vi "Build New AIM ARINC 664 Custom Device.vi"(6 "Bin File Parameter Data":path=path "Support/2FrameProperlyDefined.bin", 7 "Base System Definition File":path=path "Support/Base.nivssdf", 9 "XML File Parameter Data":path=path "Support/UDP_RX_TX_Loopback_TxRxMon.xml", 11 "Output System Definition File":path=path "Support/Scripted AIM ARINC 664.nivssdf") -> (3 "AIM ARINC 664 System Definition":path)   [LabVIEW 2020]
doc: "Overview: Demonstrates using the AIM ARINC 664 scripting API to configure the custom device by building from configuration clusters. \n\nInstructions:\n1. Run this example VI, which will create an instance of the AIM ARINC 664 Custom Device in a VeriStand system definition with a configuration matching the constants on the block diagram.\n2. (VeriStand) Optionally, you may open the Output System Definition File in VeriStand, configure the Target, and deploy the scripted system definition to perform avionics bus communications with AIM ARINC 664 hardware."
uses:
  AIM ARINC 664 Scripting Examples.lvlib
  <vilib>/addons/VeriStand Custom Device Scripting APIs/AIM ARINC 664/Scripting/AIM ARINC 664 Scripting.lvlib
  <vilib>/addons/VeriStand Custom Device Scripting APIs/AIM ARINC 664/Import/_typedefs/session_tx_generic.ctl
  <vilib>/addons/VeriStand Custom Device Scripting APIs/AIM ARINC 664/Import/AIM ARINC 664 Import.lvlib
  <vilib>/addons/VeriStand Custom Device Scripting APIs/AIM ARINC 664/Import/_typedefs/session_rx_monitor.ctl
  <vilib>/addons/VeriStand Custom Device Scripting APIs/AIM ARINC 664/Import/_typedefs/frame_tx_generic_seqNumberOffset.ctl
  <vilib>/addons/VeriStand Custom Device Scripting APIs/AIM ARINC 664/Import/_typedefs/frame_tx_generic_seqNumberInit.ctl
  <vilib>/addons/VeriStand Custom Device Scripting APIs/AIM ARINC 664/Import/_typedefs/tx_generic_setup.ctl
  <vilib>/addons/VeriStand Custom Device Scripting APIs/AIM ARINC 664/Import/_typedefs/board_setup.ctl
  NationalInstruments.VeriStand.SystemDefinitionAPI
  <vilib>/addons/VeriStand Custom Device Scripting APIs/AIM ARINC 664/Shared/Encoding (Arinc664).ctl
  <vilib>/addons/VeriStand Custom Device Scripting APIs/AIM ARINC 664/Import/_typedefs/frame_parameter_definition.ctl
  <vilib>/addons/VeriStand Custom Device Scripting APIs/AIM ARINC 664/Import/_typedefs/frame_parameter.ctl
  <vilib>/addons/VeriStand Custom Device Scripting APIs/AIM ARINC 664/Import/_typedefs/frame_tx_generic.ctl
panel:
  # "Overview: Demonstrates using the AIM ARINC 664 scripting API to configure the custom device by building from configuration clusters. \n\nInstructions:\n1. Run this example VI, which will create an instance of the AIM ARINC 664 Custom Device in a VeriStand system definition with a configuration matching the constants on the block diagram.\n2. (VeriStand) Optionally, you may open the Output System Definition File in VeriStand, configure the Target, and deploy the scripted system definition to perform avionics bus communications with AIM ARINC 664 hardware."
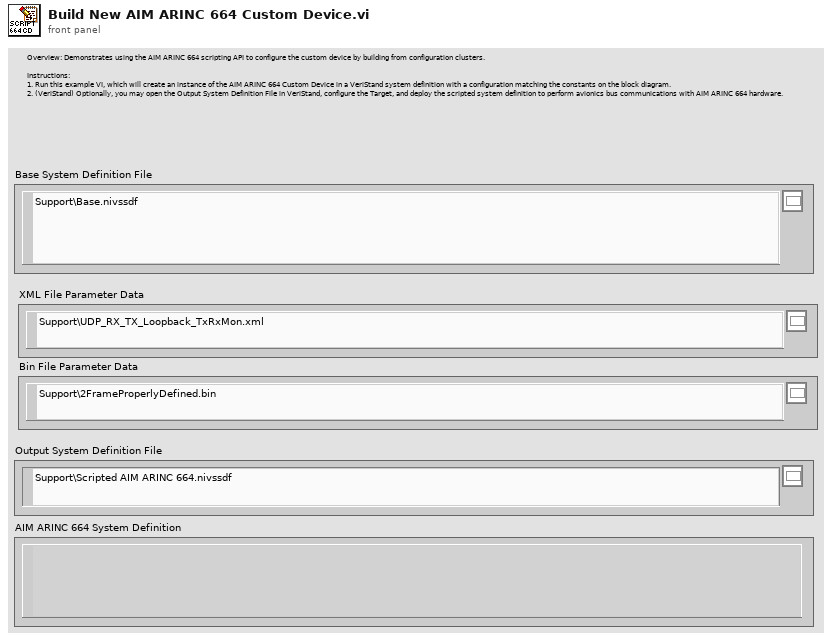
[diagram p1: front panel]
types:
  T1 = typedef "AIM ARINC 664 Import.lvlib/board_setup.ctl" = cluster{"boardId":u32, "portSpeed":u32, "portConfig":u32}
  T2 = typedef "AIM ARINC 664 Import.lvlib/session_rx_monitor.ctl" = cluster{"DefaultCronoMode":u32, "GlbMonBufferSizeIn":u32, "CaptureMode":u32, "MaxFileSizeMB":u32, "Strobe":u32, "TriggerPosition":u32}
  T3 = typedef "AIM ARINC 664 Import.lvlib/session_tx_generic.ctl" = cluster{"tx_generic_setup":T4, "Frame Headers":T5[]}
  T4 = typedef "AIM ARINC 664 Import.lvlib/tx_generic_setup.ctl" = cluster{"QueueSizeIn":u32, "Count":i32, "StartMode":i32}
  T5 = typedef "AIM ARINC 664 Import.lvlib/frame_tx_generic.ctl" = cluster{"FrameID":string, "PayloadID":string, "Frame header":cluster{"FrameStartMode":i32, "InterFrameGap":i32, "PacketGroupWaitTime":i32, "NetSelect":u32, "PayloadBufferMode":i32, "PayloadGenerationMode":i32, "PhysErrorInjection":i32, "PreambleCount":i32, "SequenceNumberInit":T6, "SequenceNumberOffset":T7, "Skew":i32}, "Parameters":T8[]}
  T6 = typedef "AIM ARINC 664 Import.lvlib/frame_tx_generic_seqNumberInit.ctl" = i32
  T7 = typedef "AIM ARINC 664 Import.lvlib/frame_tx_generic_seqNumberOffset.ctl" = i32
  T8 = typedef "AIM ARINC 664 Import.lvlib/frame_parameter.ctl" = cluster{"name":string, "default value":dbl, "unit":string, "Parameter":T9}
  T9 = typedef "AIM ARINC 664 Import.lvlib/frame_parameter_definition.ctl" = cluster{"start index":i32, "size":i32, "encoding":T10, "signed":bool, "scale multiplier":dbl, "scale offset":dbl}
  T10 = typedef "Encoding (Arinc664).ctl" = u16
  T11 = typedef "Custom Device API.lvlib/Custom Device Item Ref.ctl" = u64
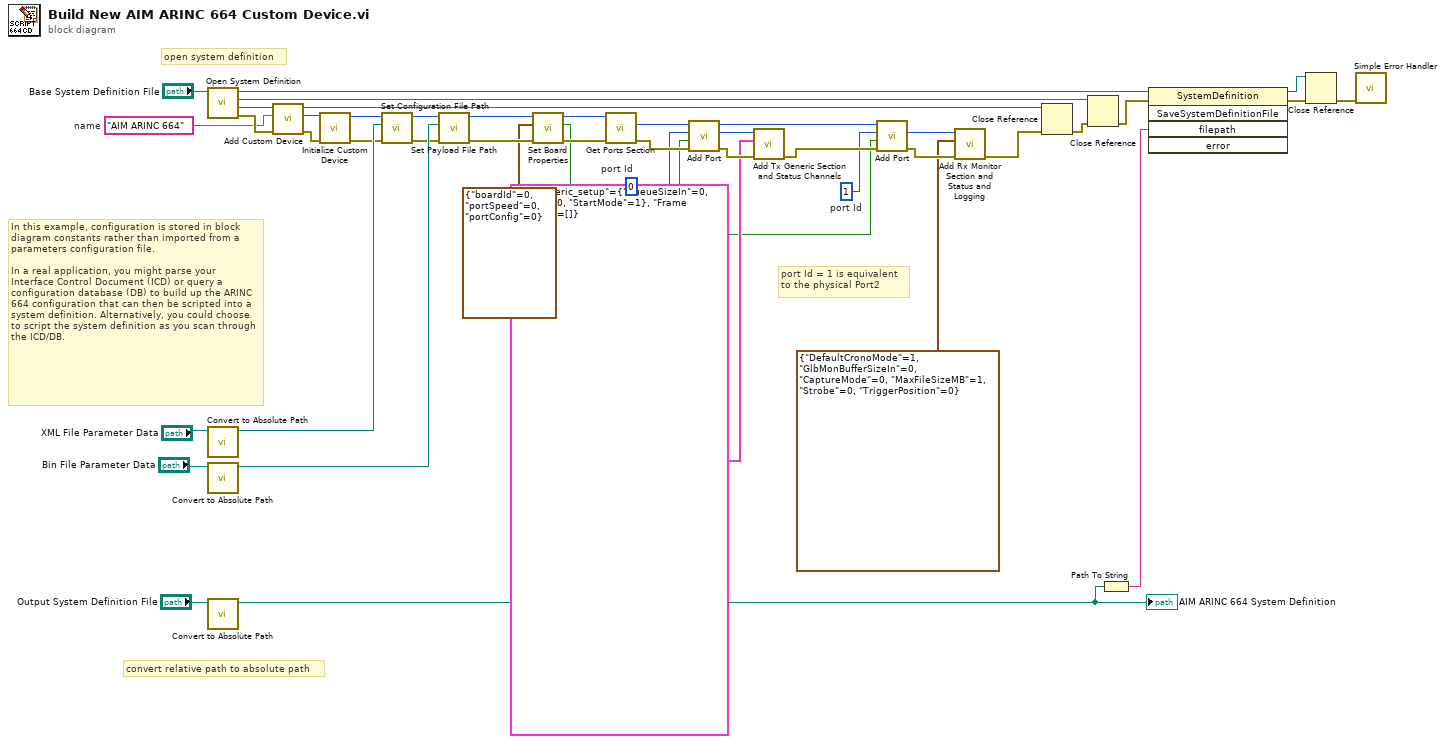
[diagram p0: block diagram]
diagram:
  w2 = u32 1  # port Id
  w9 = u32 0  # port Id
  w31 = "AIM ARINC 664"  # name
  # "port Id = 1 is equivalent \nto the physical Port2"
  # "port Id = 0 is equivalent \nto the physical Port1"
  # "open system definition"
  # "convert relative path to absolute path"
  # "In this example, configuration is stored in block diagram constants rather than imported from a parameters configuration file.\n\nIn a real application, you might parse your Interface Control Document (ICD) or query a configuration database (DB) to build up the ARINC 664 configuration that can then be scripted into a system definition. Alternatively, you could choose to script the system definition as you scan through the ICD/DB."
  # "8."
  n1 = call "Open System Definition.vi"("system definition file"="Base System Definition File") -> ("error out"=w34:errorcluster, "target"=w33:refnum<k24>, "root"=w36:refnum<k24>, "system definition"=w37:refnum<k24>)  [unwired: 7 in]
  n2 = call "Convert to Absolute Path.vi"("system definition file"="XML File Parameter Data") -> ("absolute path"=w15:path)  [unwired: 10 in]
  n3 = call "Convert to Absolute Path.vi"("system definition file"="Bin File Parameter Data") -> ("absolute path"=w14:path)  [unwired: 10 in]
  n4 = call "Convert to Absolute Path.vi"("system definition file"="Output System Definition File") -> ("absolute path"=w30:path)  [unwired: 10 in]
  "AIM ARINC 664 System Definition" <- w30
  n5 = call <vilib>:"Add Custom Device.vi"("error in"=w34, "name"=w31, "target in"=w33) -> ("error out"=w18:errorcluster, "custom device"=w19:T11, "target out"=w32:refnum<k24>)  [unwired: 6 in]
  n6 = call <vilib>:"Initialize Custom Device.vi"("error in"=w18, "custom device ref"=w19) -> ("error out"=w12:errorcluster, "custom device ref out"=w10:T11)  [unwired: 8 in]
  n7 = call <vilib>:"Set Configuration File Path.vi"("error in"=w12, "configuration file path"=w15, "custom device ref in"=w10) -> ("error out"=w13:errorcluster, "custom device ref out"=w11:T11)  [unwired: 7 in]
  n8 = call <vilib>:"Set Payload File Path.vi"("error in"=w13, "frame array file path"=w14, "custom device ref in"=w11) -> ("error out"=w6:errorcluster, "custom device ref out out"=w8:T11)  [unwired: 7 in]
  n9 = call <vilib>:"Set Board Properties.vi"("error in"=w6, "board setup"=T1 {"boardId"=0, "portSpeed"=0, "portConfig"=0}, "custom device ref in"=w8) -> ("error out"=w5:errorcluster, "redundant?"=w3:bool, "custom device ref out"=w7:T11)  [unwired: 6 in]
  n10 = call <vilib>:"Get Ports Section.vi"("error in"=w5, "custom device ref"=w7) -> ("error out"=w23:errorcluster, "ports ref out"=w24:T11)  [unwired: 6 in, 2 out]
  n11 = call <vilib>:"Add Port.vi"("error in"=w23, "redundant ?"=w3, "port Id"=w9, "ports ref"=w24) -> ("error out"=w27:errorcluster, "port ref out"=w28:T11, "ports ref out"=w29:T11)  [unwired: 5 in]
  n12 = call <vilib>:"Add Tx Generic Section and Status Channels.vi"("error in"=w27, "Tx generic configuration"=T3 {"tx_generic_setup"={"QueueSizeIn"=0, "Count"=0, "StartMode"=1}, "Frame Headers"=[]} ("session_tx_generic"), "port ref"=w28) -> ("error out"=w17:errorcluster)  [unwired: 7 in, 1 out]
  n13 = call <vilib>:"Add Port.vi"("error in"=w17, "redundant ?"=w3, "port Id"=w2, "ports ref"=w29) -> ("error out"=w25:errorcluster, "port ref out"=w26:T11)  [unwired: 5 in, 1 out]
  n14 = call <vilib>:"Add Rx Monitor Section and Status and Logging.vi"("error in"=w25, "session_rx_monitor"=T2 {"DefaultCronoMode"=1, "GlbMonBufferSizeIn"=0, "CaptureMode"=0, "MaxFileSizeMB"=1, "Strobe"=0, "TriggerPosition"=0}, "port ref"=w26) -> ("error out"=w1:errorcluster)  [unwired: 7 in, 1 out]
  n15 = Close Reference(reference=w32, error in (no error)=w1) -> (error out=w35:errorcluster)
  n16 = Close Reference(reference=w36, error in (no error)=w35) -> (error out=w40:errorcluster)
  n17 = Path To String(path=w30) -> (string=w43:string)
  n18 = invoke class="SystemDefinition" method="SaveSystemDefinitionFile"(reference=w37, error in=w40, "filepath"=w43) -> (reference out=w41:refnum<k24>, error out=w42:errorcluster)  [unwired: 2 in, 3 out]
  n19 = Close Reference(reference=w41, error in (no error)=w42) -> (error out=w39:errorcluster)
  n20 = call <vilib>:"Simple Error Handler.vi"("error in (no error)"=w39) -> ()  [unwired: 1 in, 8 out]
